vi "LoadPicture.vi"(6 "Transparent Color":fxp<+,3,3>, 8 "error in (no error)":errorcluster, 10 "Picture Path":path, 11 "RT_Sprite in":refnum<class "RT_Sprite.lvclass">) -> (0 "error out":errorcluster, 3 "RT_Sprite out":refnum<class "RT_Sprite.lvclass">)   [LabVIEW 2019, in "RT_Game.lvlib" / "RT_Sprite.lvclass"]
uses:
  RT_Sprite.lvclass
  C:/Users/FreshBob/Dropbox/VIs/myRIO_GameConsole/RT/RT_Game/GameObject/GameObject.lvclass
  Game/Coordinate.ctl
  RT_Sprite.lvclass/RT_Sprite.ctl
  GameObject/GameObject.lvclass/GameObject.ctl
  GameObject/Write size.vi
  Game/Game.lvclass
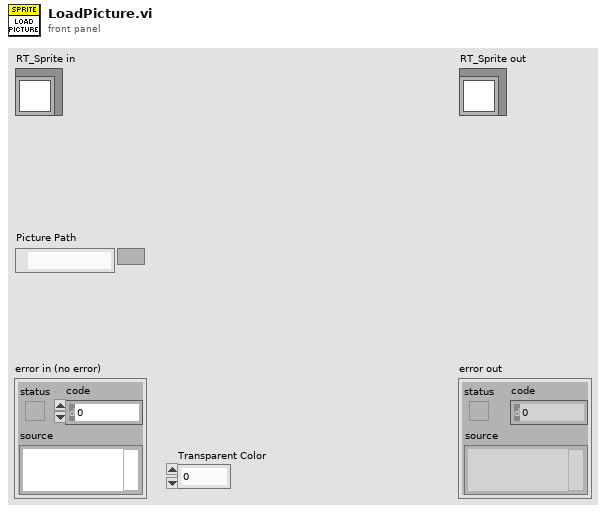
[diagram p1: front panel]
types:
  T1 = typedef "RT_Game.lvlib/Game.lvclass/Coordinate.ctl" = cluster{"x":dbl, "y":dbl}
  T2 = typedef "Color (U64)" = cluster{"Plane 3 (Blue)":u16, "Plane 2 (Green)":u16, "Plane 1 (Red)":u16, "Plane 4 (alpha)":u16}
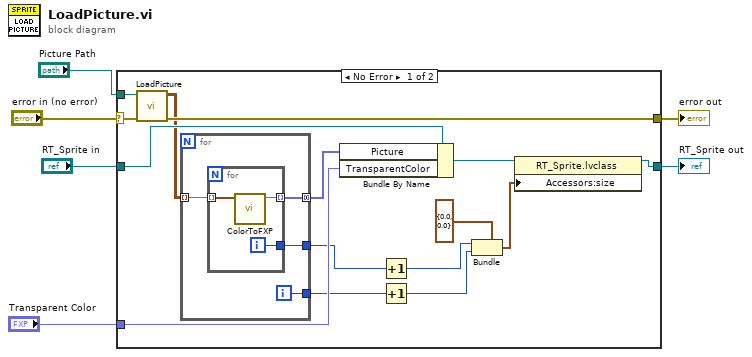
[diagram p0: block diagram]
diagram:
  n1 = case shown="No Error" "error in (no error)" {
    selector: "error in (no error)" -> [w17 w30]
    tunnel: [w16 w30] -> w5
    tunnel: [w13 w29] -> w3
    tunnel: "RT_Sprite in" -> [w21 w29]
    tunnel: "Picture Path" -> [w18 _]
    tunnel: "Transparent Color" -> [w19 _]
    frame No Error {
      n2 = call "LoadPicture.vi"("error in (no error)"=w17, "path to PNG file"=w18) -> ("error out"=w16:errorcluster, "Image Pixels (U64)"=w15:T2[][])  [unwired: 8 in]
      n3 = for {
        tunnel: w15 -> [w25] mode=indexing
        tunnel: [w24] -> w14 mode=concatenating
        tunnel: [w23] -> w9
        tunnel: [w22] -> w10
        i -> [w23]
        n4 = for {
          tunnel: w25 -> [w27] mode=indexing
          tunnel: [w26] -> w24 mode=indexing
          tunnel: [w28] -> w22
          i -> [w28]
          n5 = call "ColorToFXP.vi"("Color (U64)"=w27) -> ("Numeric"=w26:fxp<+,3,3>)  [unwired: 10 in]
        }
      }
      n6 = Bundle By Name(cluster=w21, "Picture"=w14, "TransparentColor"=w19) -> (w20:refnum<class "RT_Sprite.lvclass">)
      n7 = Increment(x=w10) -> (x+1=w8:i32)
      n8 = Increment(x=w9) -> (x+1=w7:i32)
      n9 = Bundle(cluster=T1 {"x"=0.0, "y"=0.0} ("size"), "x"=w8, "y"=w7) -> (w11:T1)
      n10 = property class="RT_Sprite.lvclass"(reference=w20, "Accessors:size"=w11) -> (reference out=w13:refnum<class "RT_Sprite.lvclass">)  [unwired: 1 in, 1 out]
    }
    frame Error {
    }
  }
  "error out" <- w5
  "RT_Sprite out" <- w3
